vi "ATF-Pump-Drive control.vi"(7 "Action":enum16{"Init", "Write", "Read"}(ring), 8 "error in":errorcluster, 11 "Loop Control In":T1) -> (0 "error Out":errorcluster, 3 "Loop Control Out":T1)   [LabVIEW 2022 SP3]
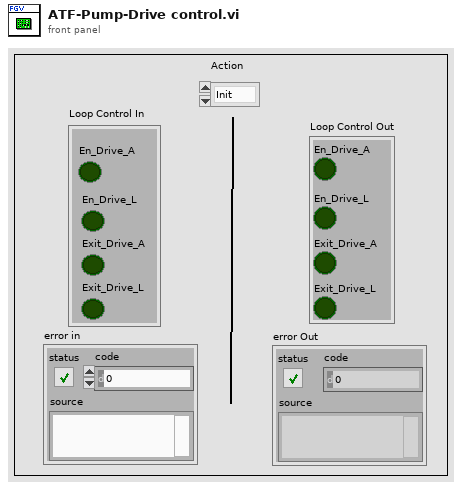
[diagram p1: front panel]
types:
  T1 = cluster{"En_Drive_A":bool, "En_Drive_L":bool, "Exit_Drive_A":bool, "Exit_Drive_L":bool}
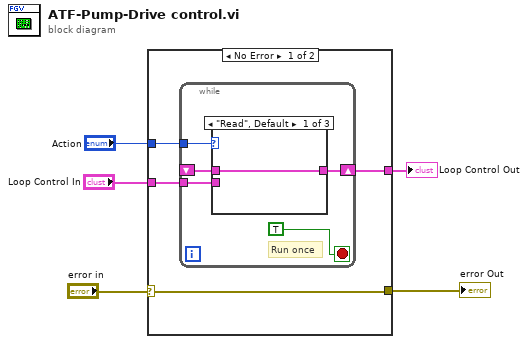
[diagram p0: block diagram]
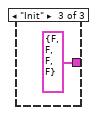
[diagram p3: hidden frame]
diagram:
  n1 = case shown="No Error" "error in" {
    selector: "error in" -> [w6 _]
    tunnel: "Action" -> [w9 _]
    tunnel: "Loop Control In" -> [w8 _]
    tunnel: [w7 _] -> w3
    tunnel: [w6 _] -> w1
    frame No Error {
      n2 = while {
        tunnel: w9 -> [w13]
        tunnel: w8 -> [w12]
        shift-right: [w11] -> w7
        shift-left: _ -> [w10]
        stop <- TRUE stop-if-true
        # "Run once"
        n3 = case shown="\"Read\", Default" w13 {
          tunnel: w12 -> [_ w16 _]
          tunnel: [w15 w16 T1 {"En_Drive_A"=FALSE, "En_Drive_L"=FALSE, "Exit_Drive_A"=FALSE, "Exit_Drive_L"=FALSE} ("Loop Control In")] -> w11
          tunnel: w10 -> [w15 _ _]
          frame "Read", Default {
          }
          frame "Write" {
          }
          frame "Init" {
          }
        }
      }
    }
    frame Error {
    }
  }
  "Loop Control Out" <- w3
  "error Out" <- w1
